vi "Helper Extension Removal2.vi"(11 "Test Case In":refnum<class "VI Tree.lvclass">) -> (0 "error out":errorcluster, 3 "Test Case Out":refnum<class "VI Tree.lvclass">)   [LabVIEW 2020, in "VI Tree.lvclass"]
uses:
  VI Tree.lvclass
  VI Tree.lvclass/VI Tree.ctl
  4993e8ee-a06a-463a-9684-69129f64d5ce.vi
  source/VI Properties Editor.lvlib
  source/SubVIs/Tree Map/Tree Map/Tree Map.lvclass
panel:
  in  "Tree":string(tree)
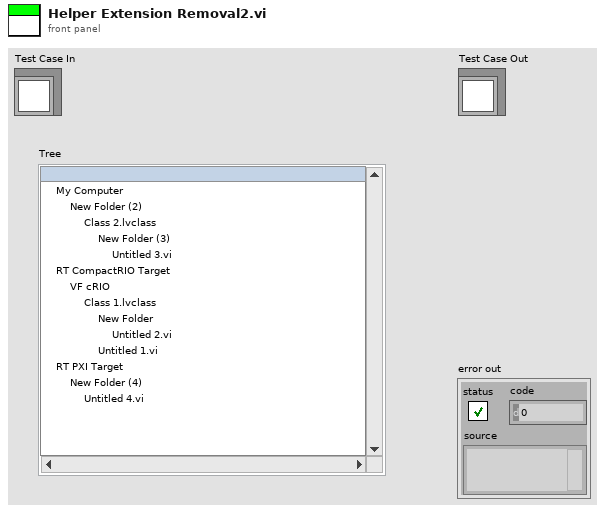
[diagram p1: front panel]
types:
  T1 = typedef "VI Properties Editor.lvlib/VI Data.ctl" = cluster{"VI":T2, "Ctl Properties":T4[], "Hierarchy":string}
  T2 = typedef "VI Properties Editor.lvlib/VI Properties.ctl" = cluster{"Name":string, "Path":path, "Type":enum32{"invalid VI type", "Standard VI", "Control VI", "Global VI", "Polymorphic VI", "Configuration VI", "SubSystem", "Facade VI", "Method VI", "Statechart Diagram VI"}, "Window Title":string, "Description":string, "Help Path":path, "Help Tag":string, "Help Web URL":string, "Use Web URL?":bool, "Custom Title?":bool, "Allow Debugging?":bool, "Reentrant?":bool, "Inlined?":bool, "Reentrancy Type":enum16{"Share clones between instances", "Preallocate clone for each instance"}, "Priority":enum32{"invalid priority", "background priority", "normal priority", "above normal priority", "high priority", "time critical priority", "subroutine"}, "Preferred Exec System":enum32{"invalid execution system", "user interface", "standard", "instrument i/o", "data acquisition", "other 1", "other 2", "same as caller"}, "Auto Error Handling?":bool, "Run When Opened?":bool, "Suspend When Called?":bool, "Conpane Img":T3}
  T3 = typedef "imagedata.ctl" = cluster{"image type":i32, "image depth":i32, "image":u8[], "mask":u8[], "colors":u32[], "Rectangle":cluster{"left":i16, "top":i16, "right":i16, "bottom":i16}}
  T4 = typedef "VI Properties Editor.lvlib/Control Properties.ctl" = cluster{"UID":i32, "Name":string, "Caption":string, "Description":string, "Tip Strip":string, "Is Indicator?":bool, "Is on ConPane?":bool}
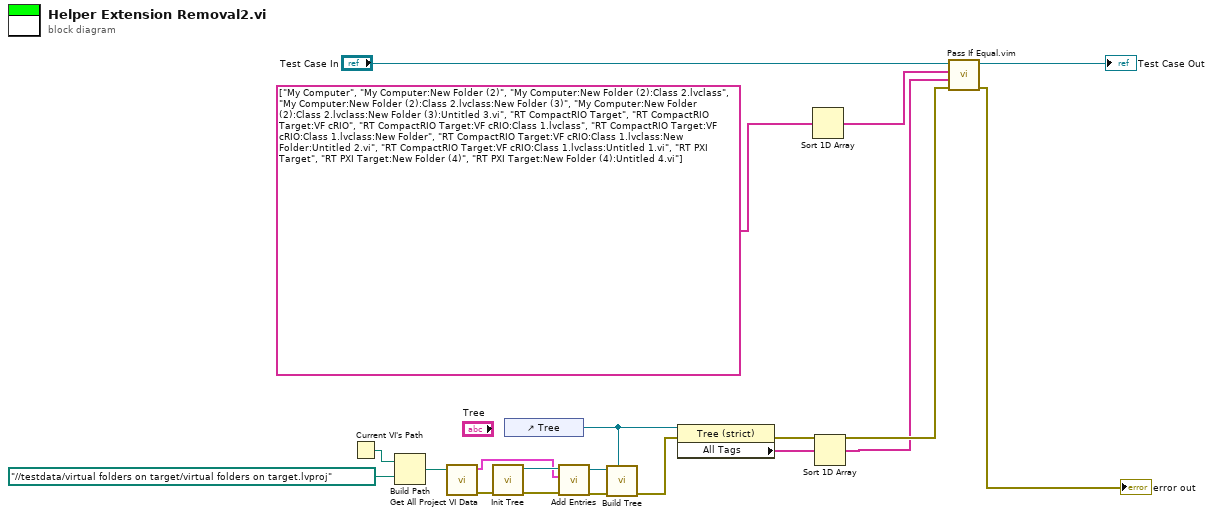
[diagram p0: block diagram]
diagram:
  n1 = Current VI's Path() -> (path=w16:path)
  n2 = Build Path(base path=w16, name or relative path=path "../../testdata/virtual folders on target/virtual folders on target.lvproj") -> (appended path=w14:path)
  n3 = call "Get All Project VI Data.vi"("Lvproj Path"=w14) -> ("error out"=w13:errorcluster, "VI Data"=w10:T1[])  [unwired: 9 in]
  n4 = call "Init Tree.vi"("error in"=w13) -> ("error out"=w12:errorcluster, "Tree Map out"=w11:refnum<class "Tree Map.lvclass">)  [unwired: 9 in]
  n5 = control-ref of="Tree"() -> (w6:refnum<vi>)
  n6 = call "Add Entries.vi"("error in"=w12, "VI Data"=w10, "Tree Map in"=w11) -> ("error out"=w9:errorcluster, "Tree Map out"=w8:refnum<class "Tree Map.lvclass">)  [unwired: 7 in]
  n7 = call "Build Tree.vi"("Tree"=w6, "error in"=w9, "Tree Map in"=w8) -> ("error out"=w7:errorcluster)  [unwired: 7 in, 1 out]
  n8 = property class="Tree (strict)"(reference=w6, error in=w7) -> (error out=w5:errorcluster, "All Tags"=w2:string[])  [unwired: 1 out]
  n9 = Sort 1D Array(array=string[] ["My Computer", "My Computer:New Folder (2)", "My Computer:New Folder (2):Class 2.lvclass", "My Computer:New Folder (2):Class 2.lvclass:New Folder (3)", "My Computer:New Folder (2):Class 2.lvclass:New Folder (3):Untitled 3.vi", "RT CompactRIO Target", "RT CompactRIO Target:VF cRIO", "RT CompactRIO Target:VF cRIO:Class 1.lvclass", "RT CompactRIO Target:VF cRIO:Class 1.lvclass:New Folder", "RT CompactRIO Target:VF cRIO:Class 1.lvclass:New Folder:Untitled 2.vi", "RT CompactRIO Target:VF cRIO:Class 1.lvclass:Untitled 1.vi", "RT PXI Target", "RT PXI Target:New Folder (4)", "RT PXI Target:New Folder (4):Untitled 4.vi"] ("All Tags")) -> (sorted array=w3:string[])
  n10 = Sort 1D Array(array=w2) -> (sorted array=w4:string[])
  n11 = call "Pass If Equal.vim"("error in (no error)"=w5, "Actual"=w4, "Expected"=w3, "LUnit Test Case In"="Test Case In") -> ("error out"=→"error out":errorcluster, "LUnit Test Case Out"=→"Test Case Out":refnum<class "VI Tree.lvclass">)  [unwired: 6 in]
